vi "SetChannelHW.vi"(8 "error in (no error)":errorcluster, 11 "BME_DG_G08 in":refnum<class "BME_DG_G08.lvclass">) -> (0 "error out":errorcluster, 3 "BME_DG_G08 out":refnum<class "BME_DG_G08.lvclass">)   [LabVIEW 2009, in "POLARIS BME DG.lvlib" / "BME_DG_G08.lvclass"]
doc: "VIs calls ModifyChnlHW.vi of a channel class for each channel containing in objChnls. ModifyChnlHW.vi calls appropriate DLL function, Set_G02_Delay, Set_GO5_Delay, Set_G05P2_Delay or Set_G08_Delay.\n\n\nauthor: Alexander Kessler, Helmholtz-Institut-Jena \nmaintainer: Alexander Kessler: alexander.kessler@uni-jena.de\n\nLast Change:\nLicense Agreement for this software:\n\nCopyright (C)\nHelmholtz-Institut-Jena\nFröbelsteg 3\n07743 Jena\nGermany\n\nContact: alexander.kessler@uni-jena.de\n\nThis program is free software; you can redistribute it and/or modify it under the terms of the GNU General Public License as published by the Free Software Foundation; either version 2 of the license, or (at your option) any later version.\n\nThis program is distributed in the hope that it will be useful, but WITHOUT ANY WARRANTY; without even the implied warranty of MERCHANTABILITY or FITNESS FOR A PARTICULAR PURPOSE. See the GNU General License for more details (http://www.gnu.org)."
uses:
  BME_DG_G08.lvclass
  BME_DG_G05P2/BME_DG_G05P2.lvclass
  POLARIS BME DG.lvlib
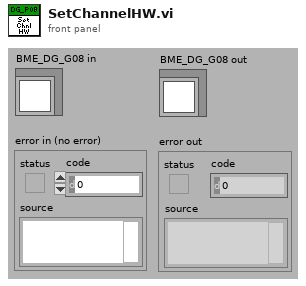
[diagram p1: front panel]
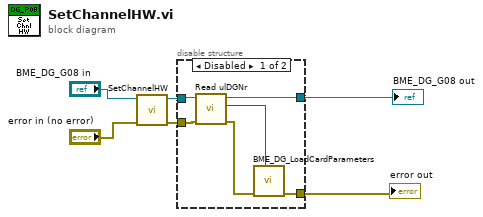
[diagram p0: block diagram]
diagram:
  n1 = call-parent "SetChannelHW.vi"("error in (no error)"="error in (no error)", "BME_DG_Base in"="BME_DG_G08 in") -> ("error out"=w2:errorcluster, "BME_DG_Base out"=w4:refnum<class "BME_DG_G08.lvclass">)  [unwired: 8 in]
  n2 = disable-structure shown="Disabled" {
    disable-tunnel: w4 -> [w12 w13]
    disable-tunnel: [w11 w13] -> w3
    disable-tunnel: w2 -> [w8 w14]
    disable-tunnel: [w9 w14] -> w1
    frame #0 {
      n3 = call-dynamic "Read ulDGNr.vi"("error in (no error)"=w8, "BME_DG_Base in"=w12) -> ("error out"=w7:errorcluster, "ulDGNr"=w10:u32, "BME_DG_Base out"=w11:refnum<class "BME_DG_G08.lvclass">)  [unwired: 6 in, 1 out]
      n4 = call "BME_DG_LoadCardParameters.vi"("DG_Number"=w10, "error in (no error)"=w7) -> ("error out"=w9:errorcluster)  [unwired: 9 in]
    }
    frame #1 {
    }
  }
  "error out" <- w1
  "BME_DG_G08 out" <- w3
